vi "Stop VIs Stream.vi"(8 "error in (no error)":errorcluster, 11 "Channel in":refnum<class "SPARC4_Channel.lvclass">) -> (0 "error out":errorcluster, 3 "Channel out":refnum<class "SPARC4_Channel.lvclass">)   [LabVIEW 2018, in "SPARC4_Channel.lvclass"]
doc: "Stop the VI responsible for communication"
uses:
  SPARC4_Channel.lvclass
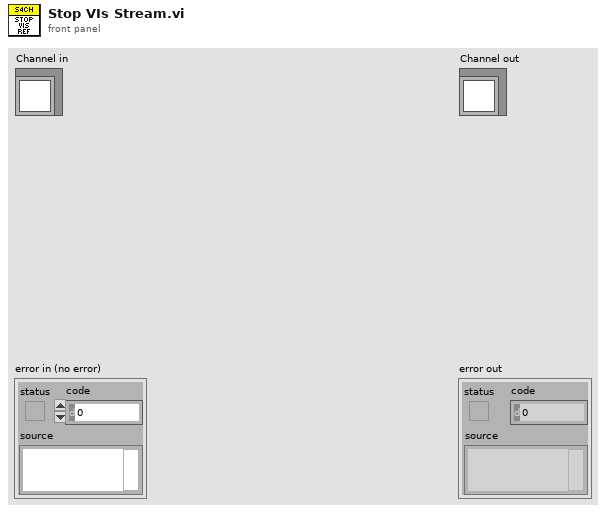
[diagram p1: front panel]
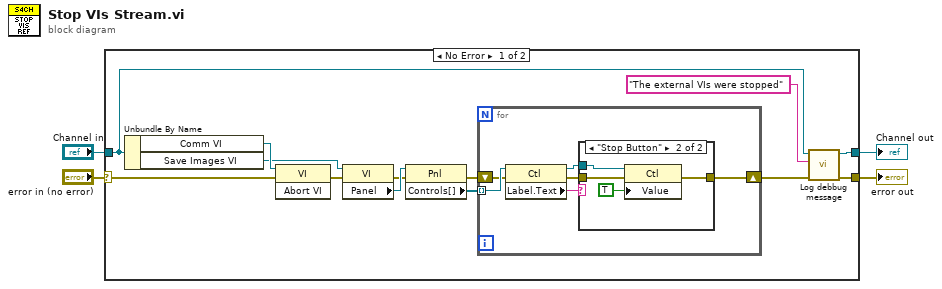
[diagram p0: block diagram]
diagram:
  n1 = case shown="No Error" "error in (no error)" {
    selector: "error in (no error)" -> [w16 w30]
    tunnel: [w8 w30] -> w3
    tunnel: [w9 w29] -> w1
    tunnel: "Channel in" -> [w6 w29]
    frame No Error {
      n2 = Unbundle By Name(w6) -> ("Comm VI"=w17:refnum<vi>, "Save Images VI"=w10:refnum<vi>)
      n3 = invoke class="VI" method="Abort VI"(reference=w17, error in=w16) -> (error out=w15:errorcluster)  [unwired: 1 in, 2 out]
      n4 = property class="VI"(reference=w10, error in=w15) -> (error out=w12:errorcluster, "Panel"=w14:refnum<vi>)  [unwired: 1 out]
      n5 = property class="Pnl"(reference=w14, error in=w12) -> (error out=w11:errorcluster, "Controls[]"=w13:refnum<vi>[])  [unwired: 1 out]
      n6 = for {
        tunnel: w13 -> [w23] mode=indexing
        shift-right: [w18] -> w7
        shift-left: w11 -> [w20]
        n7 = property class="Ctl"(reference=w23, error in=w20) -> (reference out=w21:refnum<vi>, error out=w19:errorcluster, "Label.Text"=w22:string)
        n8 = case shown="\"Stop Button\"" w22 {
          tunnel: w21 -> [_ w28]
          tunnel: w19 -> [w24 w26]
          tunnel: [w24 w25] -> w18
          frame "False", Default {
          }
          frame "Stop Button" {
            n9 = property class="Ctl"(reference=w28, error in=w26, "Value"=TRUE) -> (error out=w25:errorcluster)  [unwired: 1 out]
          }
        }
      }
      n10 = call "Log debbug message.vi"("error in (no error)"=w7, "String"="The external VIs were stopped", "Channel in"=w6) -> ("error out"=w8:errorcluster, "Channel out"=w9:refnum<class "SPARC4_Channel.lvclass">)  [unwired: 7 in]
    }
    frame Error {
    }
  }
  "error out" <- w3
  "Channel out" <- w1
